vi "ParameterParser2.vi"(1 "Parameter String":string, 2 "Controls[]":refnum<vi>[](array[refnum])) -> (0 "Array":variant[](array[variant]))   [LabVIEW 2019]
uses:
  <vilib>/Utility/Data Type/NI_Data Type.lvlib
panel:
  in  "Clust Refnum":refnum<vi>
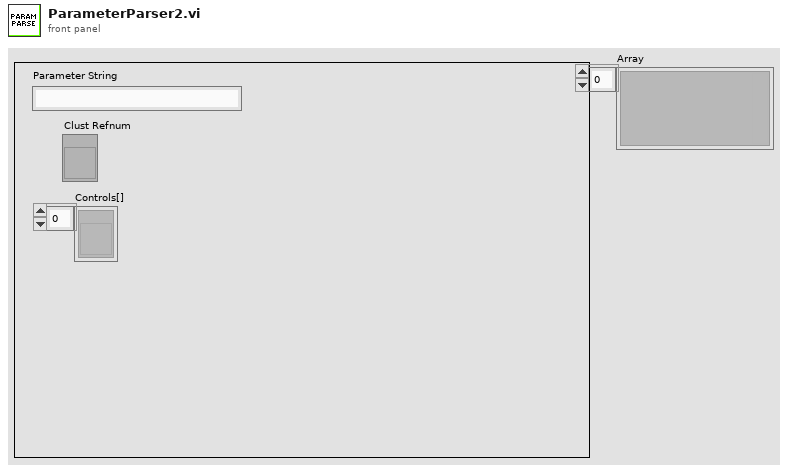
[diagram p1: front panel]
types:
  T1 = typedef "NI_Data Type.lvlib/Data Type.ctl" = enum8{"Invalid Type", "Void", "I8", "I16", "I32", "I64", "U8", "U16", "U32", "U64", "Single Float", "Double Float", "Extended Float", "Single Complex", "Double Complex", "Extended Complex", "Enum U8", "Enum U16", "Enum U32", "Enum U64", "Single Float With Unit", "Double Float With Unit", "Extended Float With Unit", "Single Complex with Unit", "Double Complex with Unit", "Extended Complex with Unit", "Boolean", "String", "Path", "Picture", "Tag", "Array", "Cluster", "Variant", "LV Variant", "Waveform", "Timestamp", "Digital Waveform", "Digital Data", "ExpressData", "Refnum", "External Data", "VI", "Poly VI", "LabVIEW Class Instance", "Fixed Point", "Set Collection", "Map Collection"}
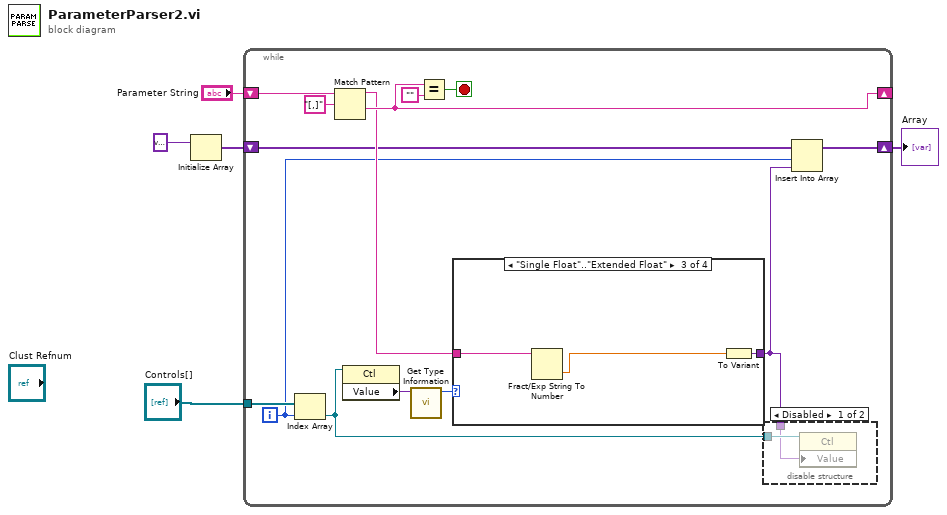
[diagram p0: block diagram]
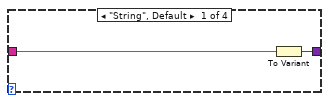
[diagram p3: hidden frame]
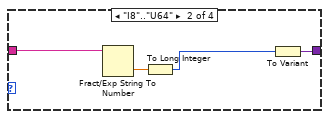
[diagram p4: hidden frame]
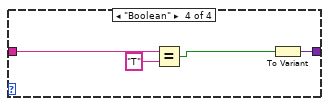
[diagram p5: hidden frame]
diagram:
  n1 = Initialize Array(variant) -> (w2:variant[])  [unwired: 1 in]
  n2 = while {
    shift-right: [w13] -> _
    shift-left: "Parameter String" -> [w18]
    tunnel: "Controls[]" -> [w11]
    shift-right: [w7] -> w1
    shift-left: w2 -> [w8]
    i -> [w6]
    stop <- w16 stop-if-true
    n3 = Index Array(array=w11, index=w6) -> (element=w15:refnum<vi>)
    n4 = Match Pattern(string=w18, regular expression="[,]") -> (before substring=w10:string, after substring=w13:string)  [unwired: 1 in, 2 out]
    n5 = property class="Ctl"(reference=w15) -> ("Value"=w14:variant)  [unwired: 1 in, 2 out]
    n6 = call <vilib>:"Get Type Information.vi"("variant"=w14) -> ("type"=w12:T1)  [unwired: 6 in, 4 out]
    n7 = Equal?(x=w13, y="") -> (x = y?=w16:bool)
    n8 = case shown="\"Single Float\"..\"Extended Float\"" w12 {
      tunnel: w10 -> [w22 w26 w30 w33]
      tunnel: [w23 w27 w29 w34] -> w9
      frame "String", Default {
        n9 = To Variant(anything=w22) -> (Variant=w23:variant)
      }
      frame "I8".."U64" {
        n10 = Fract/Exp String To Number(string=w26) -> (number=w25:dbl)  [unwired: 3 in, 1 out]
        n11 = To Long Integer(number=w25) -> (32bit integer=w24:i32)
        n12 = To Variant(anything=w24) -> (Variant=w27:variant)
      }
      frame "Single Float".."Extended Float" {
        n13 = Fract/Exp String To Number(string=w30) -> (number=w28:dbl)  [unwired: 3 in, 1 out]
        n14 = To Variant(anything=w28) -> (Variant=w29:variant)
      }
      frame "Boolean" {
        n15 = Equal?(x=w33, y="T") -> (x = y?=w31:bool)
        n16 = To Variant(anything=w31) -> (Variant=w34:variant)
      }
    }
    n17 = disable-structure shown="Disabled" {
      disable-tunnel: w15 -> [w21 _]
      disable-tunnel: w9 -> [w20 _]
      frame Disabled {
        n18 = property class="Ctl"(reference=w21, "Value"=w20) -> ()  [unwired: 1 in, 2 out]
      }
      frame Enabled {
      }
    }
    n19 = Insert Into Array(array=w8, index=w6, new element=w9) -> (w7:variant[])
  }
  "Array" <- w1
